vi "SCLN_CloseOldClients.vi"(2 "Add connection ID":refnum<k5>, 3 "Server Name":string) -> ()   [LabVIEW 2015]
uses:
  SCLN_RW_Select.ctl
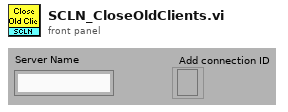
[diagram p1: front panel]
types:
  T1 = typedef "SCLN_RW_Select.ctl" = enum16{"Read", "Write"}
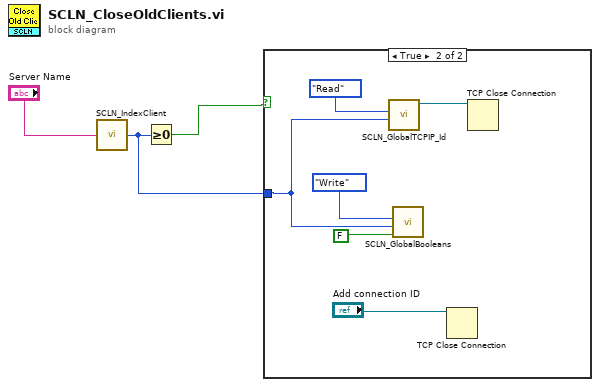
[diagram p0: block diagram]
diagram:
  n1 = call "SCLN_IndexClient.vi"("Server Name"="Server Name") -> ("Index"=w1:i32)
  n2 = Greater Or Equal To 0?(x=w1) -> (x >= 0?=w2:bool)
  n3 = case shown="True" w2 {
    tunnel: w1 -> [_ w7]
    frame False {
    }
    frame True {
      n4 = call "SCLN_GlobalTCPIP_Id.vi"("Element"=w7, "Operation"=SCLN_RW_Select."Read" ("GBL_RW")) -> ("TCPIP_Id Read"=w5:refnum<k5>)  [unwired: 2 in, 1 out]
      n5 = call "SCLN_GlobalBooleans.vi"("Write Value"=FALSE, "Element"=w7, "Operation"=SCLN_RW_Select."Write" ("GBL_RW")) -> ()  [unwired: 1 in, 2 out]
      n6 = TCP Close Connection(connection ID="Add connection ID") -> ()  [unwired: 2 in, 2 out]
      n7 = TCP Close Connection(connection ID=w5) -> ()  [unwired: 2 in, 2 out]
    }
  }
